vi "stimulus params to string gershow.vi"(7 "Stimulus cluster array":T1(array[cluster]), 8 "error in":errorcluster, 11 "Stimulus Cluster In":T2={"Stimulus Structure"=enum."Other", "Stimulant"=enum."Red Light", "Stimulant - additional detail"="", "Noise Parameters"={"Min Val"=0.0, "Noise Type"=enum."Brownian", "Max Val"=0.0, "Sigma \n(For Gaussian/Brownian)"=0.0, "Update Rate (Hz)"=0.0, "Full Scale Intensity \n(detector Watts)"=0.0, "additional string to append"="", "Other Noise Type"=""}, "Temporal Parameters"={"maximum"=0.0, "mimimum"=0.0, "period (s)"=0.0, "Temporal Pattern"=enum."Triangle", "unit"="", "additional string to append"="", "other pattern"=""}, "Spatial Parameters"={"maximum"=0.0, "mimimum"=0.0, "distance"=0.0, "Spatial Pattern"=enum."XLinear", "unit"="", "period_unit"="", "additional string to append"="", "other pattern"=""}, "Constant Parameters"={"Value"=0.0, "unit"="", "additional string to append"=""}, "Other Parameters"={"Long Description of Stimulus And Parameters"="No Stimulus Entered", "Short Description for File Name"="Nothing"}}) -> (0 "error out":errorcluster, 2 "Short String":string, 3 "Long String":string, 4 "short string array":string[](array[string]), 5 "long string array":string[](array[string]))   [LabVIEW 2021]
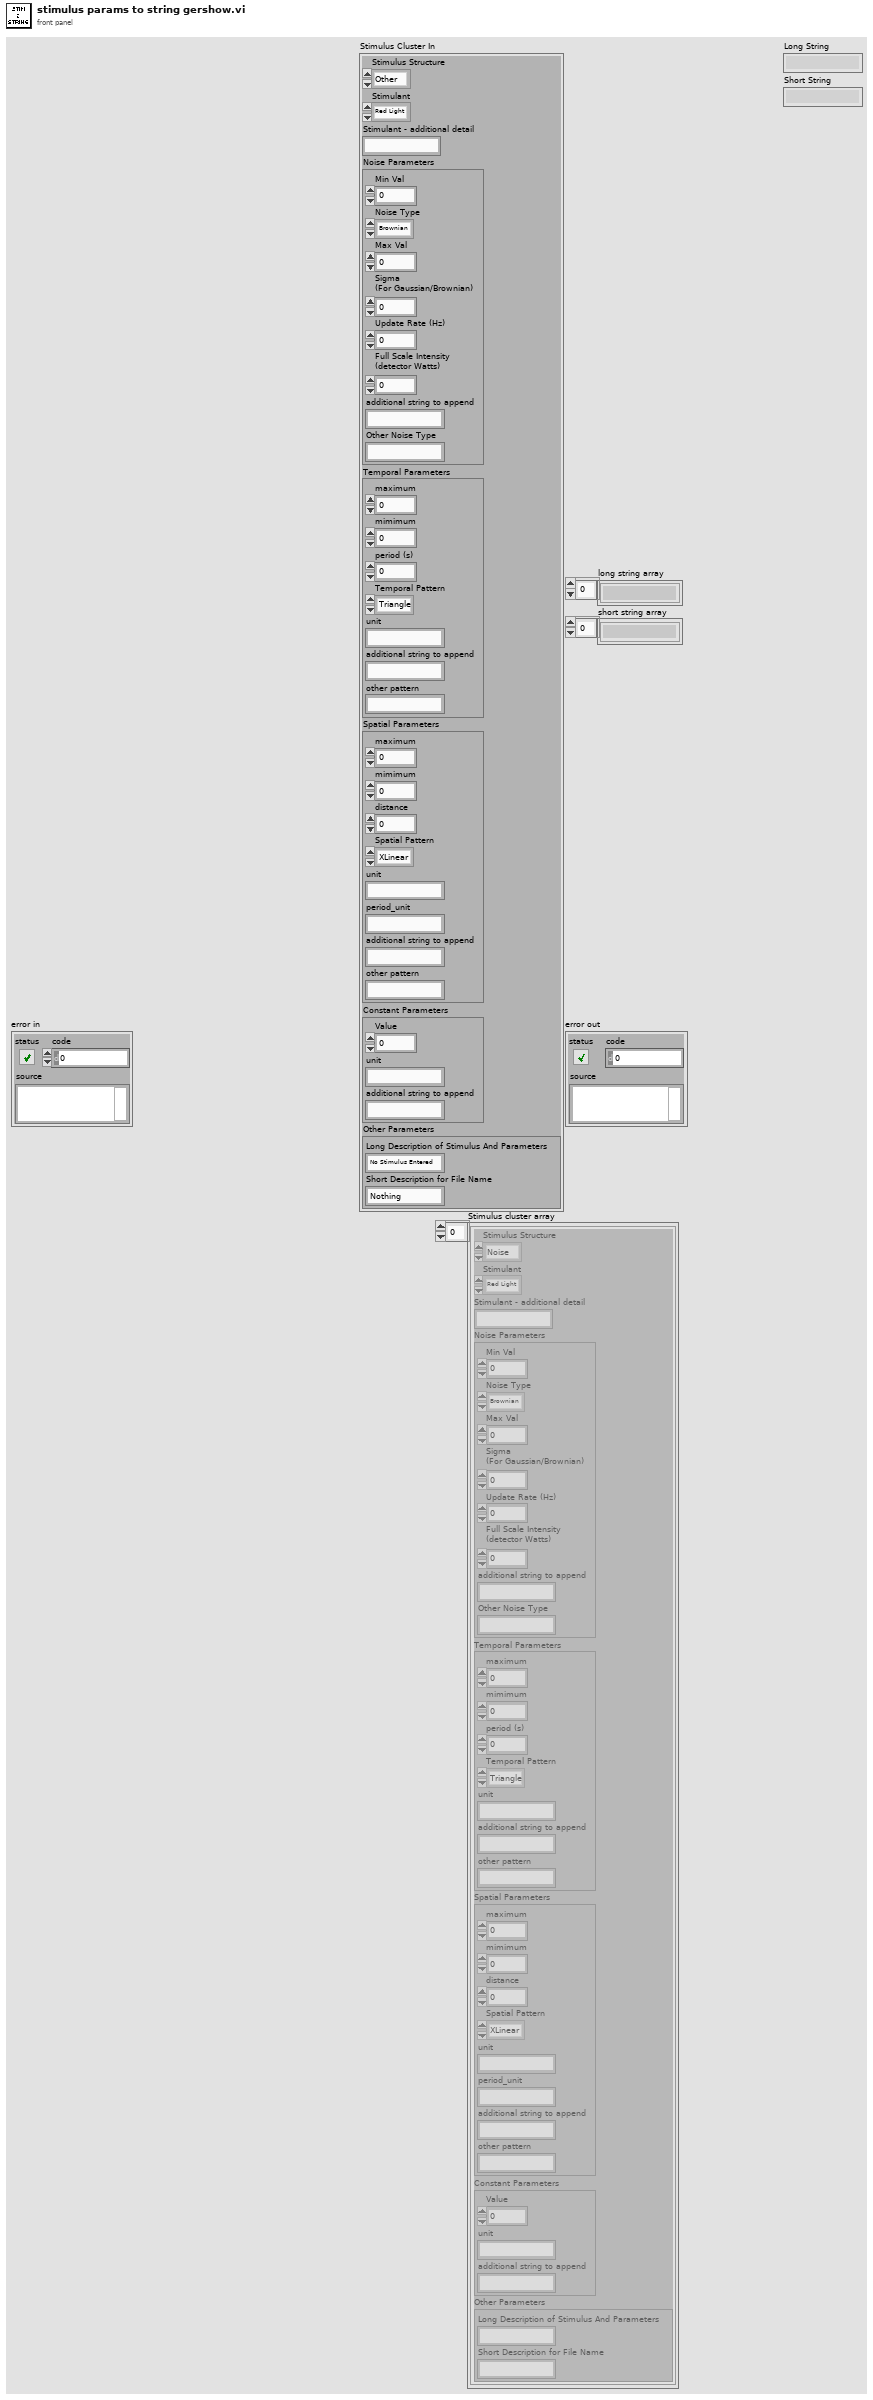
[diagram p1: front panel]
types:
  T1 = cluster{"Stimulus Structure":enum16{"Noise", "Temporal", "Spatial", "Constant", "Other"}, "Stimulant":enum16{"Red Light", "Blue Light", "Green Light", "Odor", "Temperature", "Taste", "Other"}, "Stimulant - additional detail":string, "Noise Parameters":cluster{"Min Val":dbl, "Noise Type":enum16{"Brownian", "Gaussian", "M-Sequence", "Integral of M-Sequence", "Bernoulli", "Uniform", "Other"}, "Max Val":dbl, "Sigma \n(For Gaussian/Brownian)":dbl, "Update Rate (Hz)":dbl, "Full Scale Intensity \n(detector Watts)":dbl, "additional string to append":string, "Other Noise Type":string}, "Temporal Parameters":cluster{"maximum":dbl, "mimimum":dbl, "period (s)":dbl, "Temporal Pattern":enum16{"Triangle", "Sine", "Square", "Other"}, "unit":string, "additional string to append":string, "other pattern":string}, "Spatial Parameters":cluster{"maximum":dbl, "mimimum":dbl, "distance":dbl, "Spatial Pattern":enum16{"XLinear", "YLinear", "Droplet", "Radial", "Other"}, "unit":string, "period_unit":string, "additional string to append":string, "other pattern":string}, "Constant Parameters":cluster{"Value":dbl, "unit":string, "additional string to append":string}, "Other Parameters":cluster{"Long Description of Stimulus And Parameters":string, "Short Description for File Name":string}}[]
  T2 = cluster{"Stimulus Structure":enum16{"Noise", "Temporal", "Spatial", "Constant", "Other"}, "Stimulant":enum16{"Red Light", "Blue Light", "Green Light", "Odor", "Temperature", "Taste", "Other"}, "Stimulant - additional detail":string, "Noise Parameters":cluster{"Min Val":dbl, "Noise Type":enum16{"Brownian", "Gaussian", "M-Sequence", "Integral of M-Sequence", "Bernoulli", "Uniform", "Other"}, "Max Val":dbl, "Sigma \n(For Gaussian/Brownian)":dbl, "Update Rate (Hz)":dbl, "Full Scale Intensity \n(detector Watts)":dbl, "additional string to append":string, "Other Noise Type":string}, "Temporal Parameters":cluster{"maximum":dbl, "mimimum":dbl, "period (s)":dbl, "Temporal Pattern":enum16{"Triangle", "Sine", "Square", "Other"}, "unit":string, "additional string to append":string, "other pattern":string}, "Spatial Parameters":cluster{"maximum":dbl, "mimimum":dbl, "distance":dbl, "Spatial Pattern":enum16{"XLinear", "YLinear", "Droplet", "Radial", "Other"}, "unit":string, "period_unit":string, "additional string to append":string, "other pattern":string}, "Constant Parameters":cluster{"Value":dbl, "unit":string, "additional string to append":string}, "Other Parameters":cluster{"Long Description of Stimulus And Parameters":string, "Short Description for File Name":string}}
  T3 = enum16{"Brownian", "Gaussian", "M-Sequence", "Integral of M-Sequence", "Bernoulli", "Uniform", "Other"}
  T4 = enum16{"XLinear", "YLinear", "Droplet", "Radial", "Other"}
  T5 = enum16{"Noise", "Temporal", "Spatial", "Constant", "Other"}
  T6 = enum16{"Red Light", "Blue Light", "Green Light", "Odor", "Temperature", "Taste", "Other"}
  T7 = cluster{"Min Val":dbl, "Noise Type":enum16{"Brownian", "Gaussian", "M-Sequence", "Integral of M-Sequence", "Bernoulli", "Uniform", "Other"}, "Max Val":dbl, "Sigma \n(For Gaussian/Brownian)":dbl, "Update Rate (Hz)":dbl, "Full Scale Intensity \n(detector Watts)":dbl, "additional string to append":string, "Other Noise Type":string}
  T8 = cluster{"maximum":dbl, "mimimum":dbl, "period (s)":dbl, "Temporal Pattern":enum16{"Triangle", "Sine", "Square", "Other"}, "unit":string, "additional string to append":string, "other pattern":string}
  T9 = cluster{"maximum":dbl, "mimimum":dbl, "distance":dbl, "Spatial Pattern":enum16{"XLinear", "YLinear", "Droplet", "Radial", "Other"}, "unit":string, "period_unit":string, "additional string to append":string, "other pattern":string}
  T10 = cluster{"Value":dbl, "unit":string, "additional string to append":string}
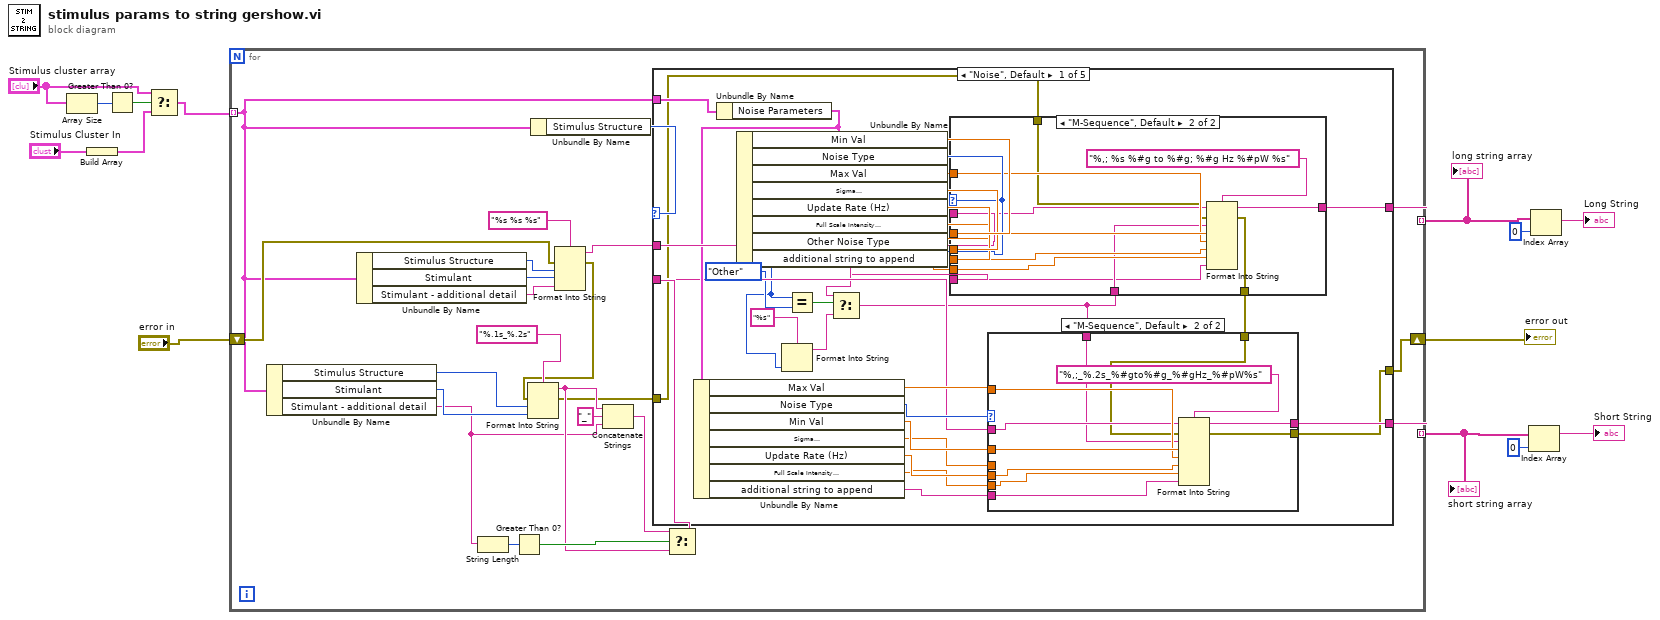
[diagram p0: block diagram]
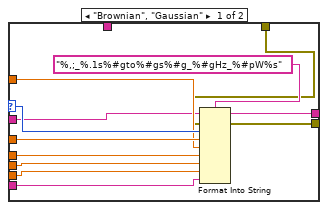
[diagram p2: hidden frame]
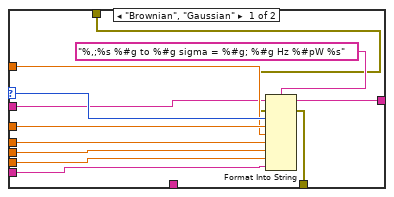
[diagram p3: hidden frame]
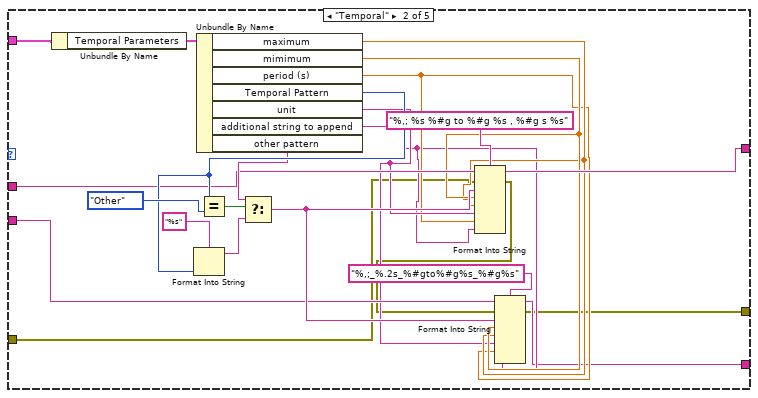
[diagram p4: hidden frame]
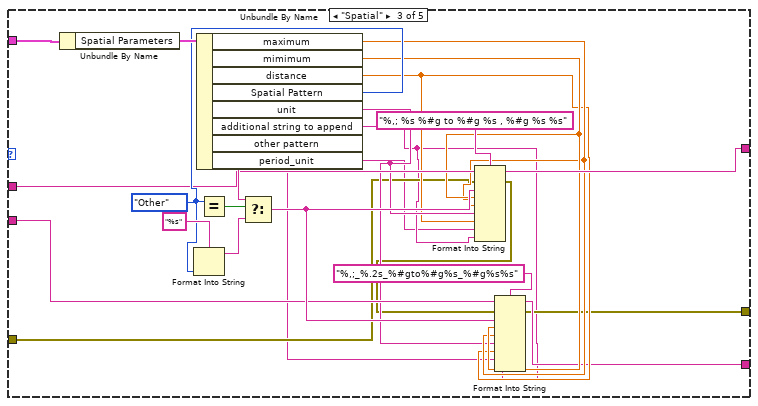
[diagram p5: hidden frame]
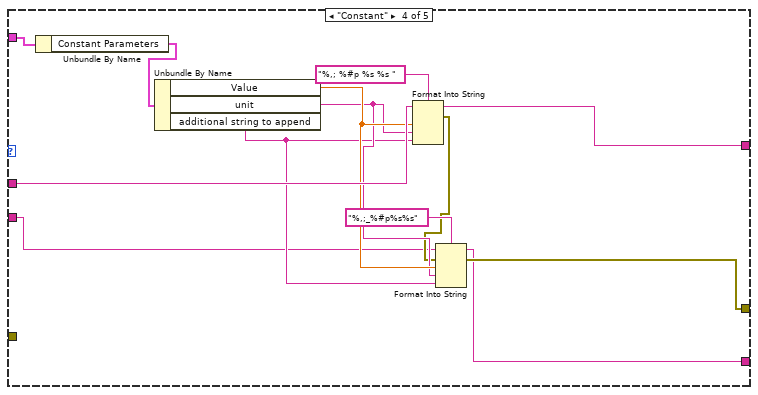
[diagram p6: hidden frame]
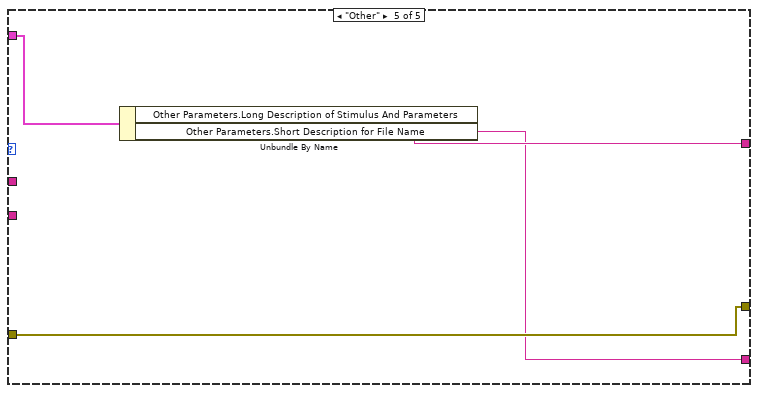
[diagram p7: hidden frame]
diagram:
  n1 = Array Size(array="Stimulus cluster array") -> (size(s)=w9:i32)
  n2 = Build Array("Stimulus Cluster In") -> (w6:T1)
  n3 = Greater Than 0?(x=w9) -> (x > 0?=w8:bool)
  n4 = Select(t="Stimulus cluster array", s=w8, f=w6) -> (s? t:f=w5:T1)
  n5 = for {
    tunnel: w5 -> [w15] mode=indexing
    tunnel: [w21] -> w13 mode=indexing
    tunnel: [w20] -> w12 mode=indexing
    shift-right: [w17] -> w11
    shift-left: "error in" -> [w16]
    n6 = Unbundle By Name(w15) -> ("Stimulus Structure"=w32:T5, "Stimulant"=w31:T6, "Stimulant - additional detail"=w25:string)
    n7 = Unbundle By Name(w15) -> ("Stimulus Structure"=w35:T5, "Stimulant"=w34:T6, "Stimulant - additional detail"=w33:string)
    n8 = String Length(string=w25) -> (length=w29:i32)
    n9 = Greater Than 0?(x=w29) -> (x > 0?=w28:bool)
    n10 = Unbundle By Name(w15) -> ("Stimulus Structure"=w37:T5)
    n11 = Format Into String(format string="%s %s %s", error in=w16, w35, w34, w33) -> (resulting string=w23:string, error out=w19:errorcluster)  [unwired: 1 in]
    n12 = Format Into String(format string="%.1s_%.2s", error in=w19, w32, w31) -> (resulting string=w26:string, error out=w18:errorcluster)  [unwired: 1 in]
    n13 = Concatenate Strings(w26, "_" ("string"), w25) -> (w24:string)
    n14 = Select(t=w24, s=w28, f=w26) -> (s? t:f=w22:string)
    n15 = case shown="\"Noise\", Default" w37 {
      tunnel: w15 -> [w66 w135 w159 w172 w175]
      tunnel: w23 -> [w60 w123 w148 w170 _]
      tunnel: w22 -> [w52 w122 w147 w162 _]
      tunnel: [w44 w116 w142 w160 w173] -> w20
      tunnel: [w43 w126 w151 w161 w174] -> w21
      tunnel: [w38 w114 w140 w163 w176] -> w17
      tunnel: w18 -> [w40 w113 w139 _ w176]
      frame "Noise", Default {
        n16 = Unbundle By Name(w66) -> ("Noise Parameters"=w59:T7)
        n17 = Unbundle By Name(w59) -> ("Max Val"=w58:dbl, "Noise Type"=w57:T3, "Min Val"=w56:dbl, "Sigma \n(For Gaussian/Brownian)"=w55:dbl, "Update Rate (Hz)"=w54:dbl, "Full Scale Intensity \n(detector Watts)"=w53:dbl, "additional string to append"=w41:string)
        n18 = Unbundle By Name(w59) -> ("Min Val"=w65:dbl, "Noise Type"=w47:T3, "Max Val"=w64:dbl, "Sigma \n(For Gaussian/Brownian)"=w63:dbl, "Update Rate (Hz)"=w62:dbl, "Full Scale Intensity \n(detector Watts)"=w61:dbl, "Other Noise Type"=w49:string, "additional string to append"=w42:string)
        n19 = Format Into String(format string="%s", w47) -> (resulting string=w46:string)  [unwired: 2 in, 1 out]
        n20 = Equal?(x=w47, y=T3."Other") -> (x = y?=w50:bool)
        n21 = Select(t=w49, s=w50, f=w46) -> (s? t:f=w45:string)
        n22 = case shown="\"M-Sequence\", Default" w47 {
          selector: w47 -> [w100 _]
          tunnel: w65 -> [w99 w111]
          tunnel: w64 -> [w98 w110]
          tunnel: w63 -> [w97 _]
          tunnel: w62 -> [w96 w109]
          tunnel: w61 -> [w95 w108]
          tunnel: w60 -> [w94 w107]
          tunnel: [w93 w106] -> w43
          tunnel: w45 -> [_ w105]
          tunnel: w42 -> [w92 w102]
          tunnel: w40 -> [w91 w104]
          tunnel: [w90 w103] -> w39
          frame "Brownian", "Gaussian" {
            n23 = Format Into String(format string="%,;%s %#g to %#g sigma = %#g; %#g Hz %#pW %s", initial string=w94, error in=w91, w100, w99, w98, w97, w96, w95, w92) -> (resulting string=w93:string, error out=w90:errorcluster)
          }
          frame "M-Sequence", Default {
            n24 = Format Into String(format string="%,; %s %#g to %#g; %#g Hz %#pW %s", initial string=w107, error in=w104, w105, w111, w110, w109, w108, w102) -> (resulting string=w106:string, error out=w103:errorcluster)
          }
        }
        n25 = case shown="\"M-Sequence\", Default" w57 {
          selector: w57 -> [w77 _]
          tunnel: w56 -> [w76 w88]
          tunnel: w58 -> [w75 w87]
          tunnel: w55 -> [w74 _]
          tunnel: w54 -> [w73 w86]
          tunnel: w53 -> [w72 w85]
          tunnel: w52 -> [w71 w84]
          tunnel: [w70 w83] -> w44
          tunnel: w45 -> [_ w82]
          tunnel: w41 -> [w69 w79]
          tunnel: w39 -> [w68 w81]
          tunnel: [w67 w80] -> w38
          frame "Brownian", "Gaussian" {
            n26 = Format Into String(format string="%,;_%.1s%#gto%#gs%#g_%#gHz_%#pW%s", initial string=w71, error in=w68, w77, w76, w75, w74, w73, w72, w69) -> (resulting string=w70:string, error out=w67:errorcluster)
          }
          frame "M-Sequence", Default {
            n27 = Format Into String(format string="%,;_%.2s_%#gto%#g_%#gHz_%#pW%s", initial string=w84, error in=w81, w82, w88, w87, w86, w85, w79) -> (resulting string=w83:string, error out=w80:errorcluster)
          }
        }
      }
      frame "Temporal" {
        n28 = Unbundle By Name(w135) -> ("Temporal Parameters"=w134:T8)
        n29 = Unbundle By Name(w134) -> ("maximum"=w120:dbl, "mimimum"=w121:dbl, "period (s)"=w118:dbl, "Temporal Pattern"=w129:enum16{"Triangle", "Sine", "Square", "Other"}, "unit"=w119:string, "additional string to append"=w117:string, "other pattern"=w128:string)
        n30 = Format Into String(format string="%s", w129) -> (resulting string=w131:string)  [unwired: 2 in, 1 out]
        n31 = Equal?(x=w129, y=enum16{"Triangle", "Sine", "Square", "Other"}."Other") -> (x = y?=w133:bool)
        n32 = Select(t=w128, s=w133, f=w131) -> (s? t:f=w124:string)
        n33 = Format Into String(format string="%,; %s %#g to %#g %s , %#g s %s", initial string=w123, error in=w113, w124, w121, w120, w119, w118, w117) -> (resulting string=w126:string, error out=w115:errorcluster)
        n34 = Format Into String(format string="%,;_%.2s_%#gto%#g%s_%#g%s", initial string=w122, error in=w115, w124, w121, w120, w119, w118, w117) -> (resulting string=w116:string, error out=w114:errorcluster)
      }
      frame "Spatial" {
        n35 = Unbundle By Name(w159) -> ("Spatial Parameters"=w158:T9)
        n36 = Unbundle By Name(w158) -> ("maximum"=w145:dbl, "mimimum"=w146:dbl, "distance"=w143:dbl, "Spatial Pattern"=w154:T4, "unit"=w144:string, "additional string to append"=w138:string, "other pattern"=w153:string, "period_unit"=w137:string)
        n37 = Format Into String(format string="%s", w154) -> (resulting string=w155:string)  [unwired: 2 in, 1 out]
        n38 = Equal?(x=w154, y=T4."Other") -> (x = y?=w157:bool)
        n39 = Select(t=w153, s=w157, f=w155) -> (s? t:f=w149:string)
        n40 = Format Into String(format string="%,; %s %#g to %#g %s , %#g %s %s", initial string=w148, error in=w139, w149, w146, w145, w144, w143, w137, w138) -> (resulting string=w151:string, error out=w141:errorcluster)
        n41 = Format Into String(format string="%,;_%.2s_%#gto%#g%s_%#g%s%s", initial string=w147, error in=w141, w149, w146, w145, w144, w143, w137, w138) -> (resulting string=w142:string, error out=w140:errorcluster)
      }
      frame "Constant" {
        n42 = Unbundle By Name(w172) -> ("Constant Parameters"=w171:T10)
        n43 = Unbundle By Name(w171) -> ("Value"=w167:dbl, "unit"=w166:string, "additional string to append"=w165:string)
        n44 = Format Into String(format string="%,; %#p %s %s ", initial string=w170, w167, w166, w165) -> (resulting string=w161:string, error out=w164:errorcluster)  [unwired: 1 in]
        n45 = Format Into String(format string="%,;_%#p%s%s", initial string=w162, error in=w164, w167, w166, w165) -> (resulting string=w160:string, error out=w163:errorcluster)
      }
      frame "Other" {
        n46 = Unbundle By Name(w175) -> ("Other Parameters.Long Description of Stimulus And Parameters"=w174:string, "Other Parameters.Short Description for File Name"=w173:string)
      }
    }
  }
  "error out" <- w11
  "long string array" <- w13
  "short string array" <- w12
  n47 = Index Array(array=w12, index=0) -> (element=→"Short String":string)
  n48 = Index Array(array=w13, index=0) -> (element=→"Long String":string)
